vi "Control_Panel_Globals.vi"() -> ()   [LabVIEW 2019]
panel:
  in  "Control_Panel":string="Control_Panel"
  in  "Control_Panel_Execute_Ref":string="Control_Panel_Execute_Ref"
  in  "Control_Panel_Set_Ref":string="Control_Panel_Set_Ref"
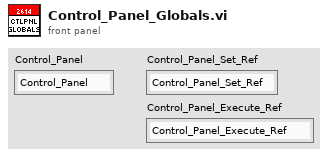
[diagram p1: front panel]
diagram:
